vi "test_Copy LogFile from Windows.vi"(8 "error in (no error)":errorcluster, 11 "TestCase in":refnum<class "Telemetry System Tests.lvclass">) -> (0 "error out":errorcluster, 3 "TestCase out":refnum<class "Telemetry System Tests.lvclass">)   [LabVIEW 2019]
uses:
  Telemetry System Tests.lvclass
  4cf6fdd8-95a5-41c0-8a99-f2e6392f4f64.vi
  <vilib>/addons/_JKI Toolkits/VI Tester/TestCase.llb/TestCase.lvclass
  TLCD Test/TLCD Test.lvclass
  C:/Program Files (x86)/National Instruments/LabVIEW 2019/vi.lib/addons/_JKI Toolkits/VI Tester/TestCase.llb/TestCase.lvclass
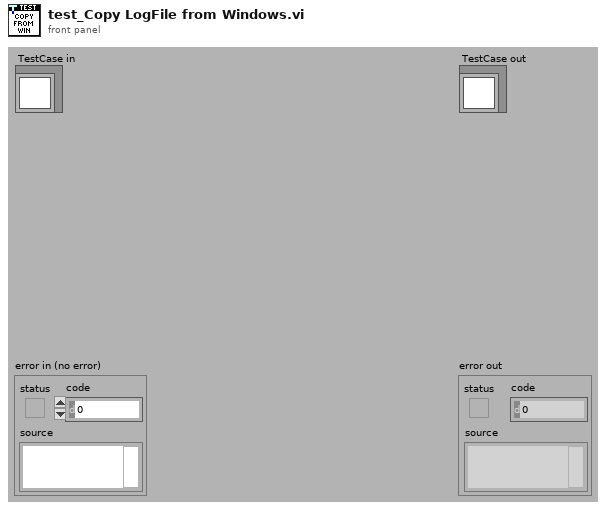
[diagram p1: front panel]
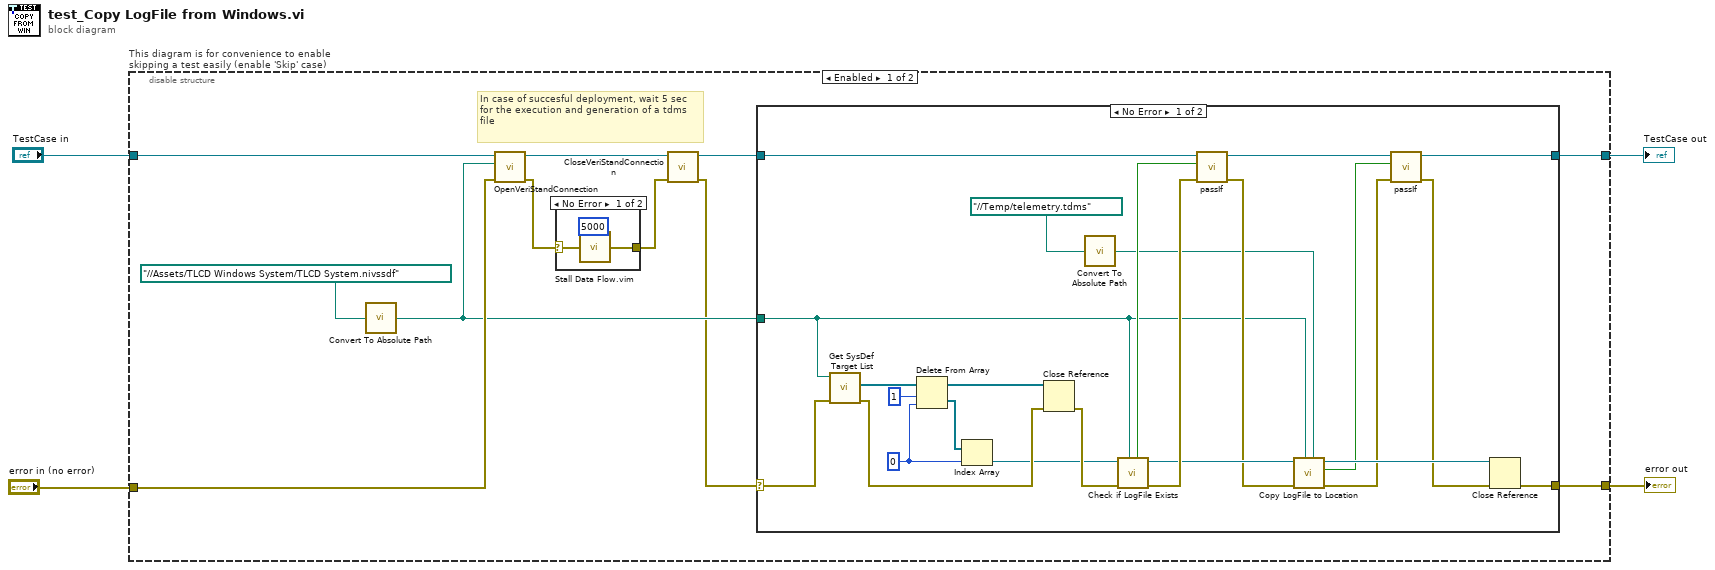
[diagram p0: block diagram]
diagram:
  n1 = disable-structure "This diagram is for convenience to enable skipping a test easily (enable 'Skip' case)" shown="Enabled" {
    disable-tunnel: "TestCase in" -> [w9 w49]
    disable-tunnel: [w13 w47] -> w1
    disable-tunnel: [w14 w48] -> w3
    disable-tunnel: "error in (no error)" -> [w7 w46]
    frame Enabled {
      # "In case of succesful deployment, wait 5 sec for the execution and generation of a tdms file"
      n2 = call "Convert To Absolute Path.vi"("System Definition File Path"=path "../../Assets/TLCD Windows System/TLCD System.nivssdf" ("relative base path")) -> ("Absolute path"=w6:path)
      n3 = call-dynamic "OpenVeriStandConnection.vi"("error in (no error)"=w7, "System Definition File"=w6, "VeriStand Test Case in"=w9) -> ("error out"=w11:errorcluster, "VeriStand Test Case out"=w12:refnum<class "Telemetry System Tests.lvclass">)  [unwired: 6 in, 1 out]
      n4 = case shown="No Error" w11 {
        selector: w11 -> [w44 w45]
        tunnel: [w42 w45] -> w10
        frame No Error {
          n5 = call "Stall Data Flow.vim"("value in"=w44, "milliseconds to wait"=u32 5000) -> ("value out"=w42:errorcluster)  [unwired: 1 out]
        }
        frame Error {
        }
      }
      n6 = call-dynamic "CloseVeriStandConnection.vi"("error in (no error)"=w10, "VeriStand Test Case in"=w12) -> ("error out"=w5:errorcluster, "VeriStand Test Case out"=w8:refnum<class "Telemetry System Tests.lvclass">)  [unwired: 8 in]
      n7 = case shown="No Error" w5 {
        selector: w5 -> [w21 w41]
        tunnel: [w39 w41] -> w14
        tunnel: [w19 w40] -> w13
        tunnel: w8 -> [w23 w40]
        tunnel: w6 -> [w22 _]
        frame No Error {
          w35 = 0 ("index")
          n8 = call "Get SysDef Target List.vi"("error in (no error)"=w21, "System Definition Path"=w22) -> ("error out"=w33:errorcluster, "Target List"=w38:refnum<k24>[])  [unwired: 8 in]
          n9 = Delete From Array(array=w38, length=1, index=w35) -> (deleted portion=w36:refnum<k24>[], array with subset deleted=w34:refnum<k24>[])
          n10 = Index Array(array=w36, index=w35) -> (element=w31:refnum<k24>)
          n11 = Close Reference(reference=w34, error in (no error)=w33) -> (error out=w32:errorcluster)
          n12 = call "Convert To Absolute Path.vi"("System Definition File Path"=path "../../Temp/telemetry.tdms" ("relative base path")) -> ("Absolute path"=w24:path)
          n13 = call "Check if LogFile Exists.vi"("System Definition Path"=w22, "error in (no error)"=w32, "Target Refnum in"=w31) -> ("error out"=w30:errorcluster, "Target Refnum out"=w28:refnum<k24>, "LogFile Exists?"=w29:bool)  [unwired: 6 in]
          n14 = call-dynamic "passIf.vi"("error in (no error)"=w30, "pass"=w29, "TestCase in"=w23) -> ("error out"=w27:errorcluster, "TestCase out"=w20:refnum<class "Telemetry System Tests.lvclass">)  [unwired: 7 in]
          n15 = call "Copy LogFile to Location.vi"("Local Save path"=w24, "System Definition Path"=w22, "error in (no error)"=w27, "Target Refnum in"=w28) -> ("error out"=w17:errorcluster, "File Succesfuly copied"=w18:bool, "Target Refnum out"=w26:refnum<k24>)  [unwired: 5 in]
          n16 = call-dynamic "passIf.vi"("error in (no error)"=w17, "pass"=w18, "TestCase in"=w20) -> ("error out"=w16:errorcluster, "TestCase out"=w19:refnum<class "Telemetry System Tests.lvclass">)  [unwired: 7 in]
          n17 = Close Reference(reference=w26, error in (no error)=w16) -> (error out=w39:errorcluster)
        }
        frame Error {
        }
      }
    }
    frame Disabled {
      # "skip test result while test is under development"
      n18 = call <vilib>:"skip.vi"("error in (no error)"=w46, "TestCase in"=w49) -> ("error out"=w48:errorcluster, "TestCase out"=w47:refnum<class "Telemetry System Tests.lvclass">)  [unwired: 8 in]
    }
  }
  "error out" <- w3
  "TestCase out" <- w1
